vi "Enable or Disable Button.vi"(8 "Error In":errorcluster, 10 "Have All Errors Been Read?":bool, 11 "Mark All Errors As Read Button Reference":refnum<vi>) -> (0 "Error Out":errorcluster)   [LabVIEW 2023, in "Error Manager.lvlib" / "Mark All Errors As Read Button.lvclass"]
doc: "This VI determines whether the \"Mark All Errors As Read\" button should be enabled or disabled and greyed out. The button should be enabled only when there are one or more unread errors. The button should be disabled and greyed out when all errors are read."
uses:
  Mark All Errors As Read Button.lvclass
  Mark All Errors As Read Button.lvclass/Mark All Errors As Read Button.ctl
panel:
  # "Development\nControls or indicators that are useful for development or testing, but which are not outputs of the VI."
  # "Input\nInputs to the VI"
  # "Output\nOutputs of the VI"
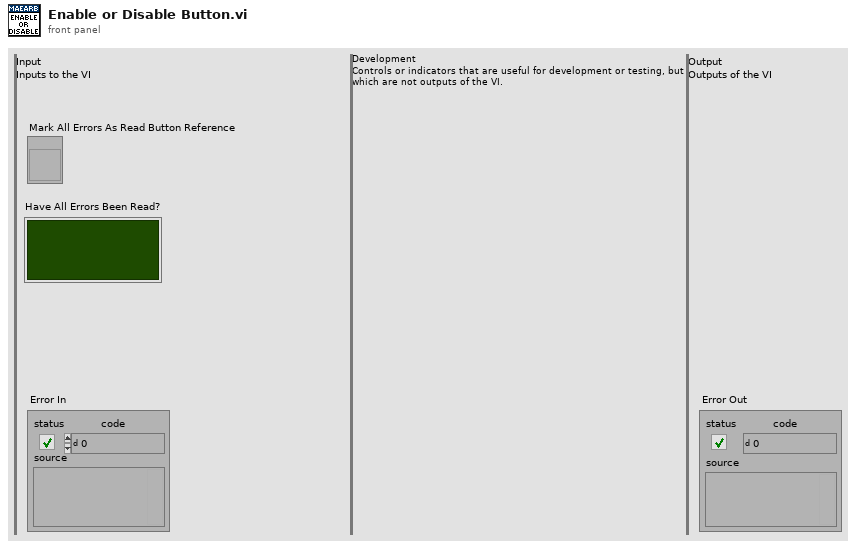
[diagram p1: front panel]
types:
  T1 = enum8{"Enabled", "Disabled", "Disabled and Grayed Out"}
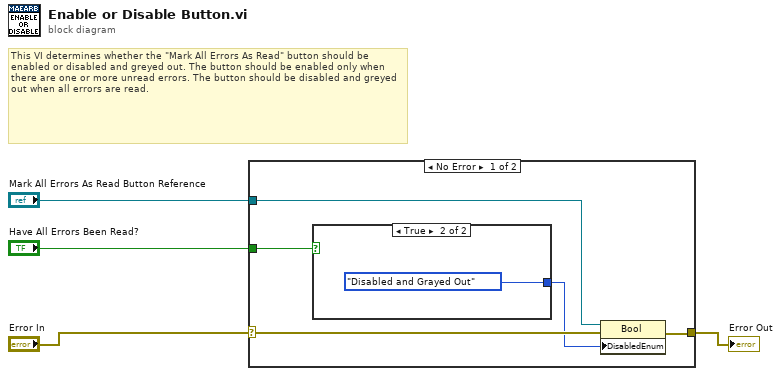
[diagram p0: block diagram]
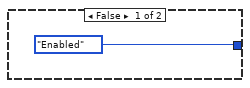
[diagram p2: hidden frame]
diagram:
  # "This VI determines whether the \"Mark All Errors As Read\" button should be enabled or disabled and greyed out. The button should be enabled only when there are one or more unread errors. The button should be disabled and greyed out when all errors are read."
  n1 = case shown="No Error" "Error In" {
    selector: "Error In" -> [w9 w12]
    tunnel: [w8 w12] -> w3
    tunnel: "Mark All Errors As Read Button Reference" -> [w7 _]
    tunnel: "Have All Errors Been Read?" -> [w6 _]
    frame No Error {
      n2 = case shown="True" w6 {
        tunnel: [T1."Enabled" ("Disabled") T1."Disabled and Grayed Out" ("Disabled")] -> w5
        frame False {
        }
        frame True {
        }
      }
      n3 = property class="Bool"(reference=w7, error in=w9, "DisabledEnum"=w5) -> (error out=w8:errorcluster)  [unwired: 1 out]
    }
    frame Error {
    }
  }
  "Error Out" <- w3
